vi "Destroy.vi"(8 "error in (no error)":errorcluster, 10 "Wait until done?":bool, 11 "InstrPtr in":refnum<class "InstrPtr.lvclass">) -> (0 "error out":errorcluster, 3 "final Instrument":refnum<class "Instrument.lvclass">)   [LabVIEW 2009, in "InstrPtr.lvclass"]
doc: "Finalizes and destroys this Instrument pointer. You can optionally block if some other process still has a handle."
uses:
  InstrPtr.lvclass
  Instrument/Instrument.lvclass
  InstrPtr.lvclass/InstrPtr.ctl
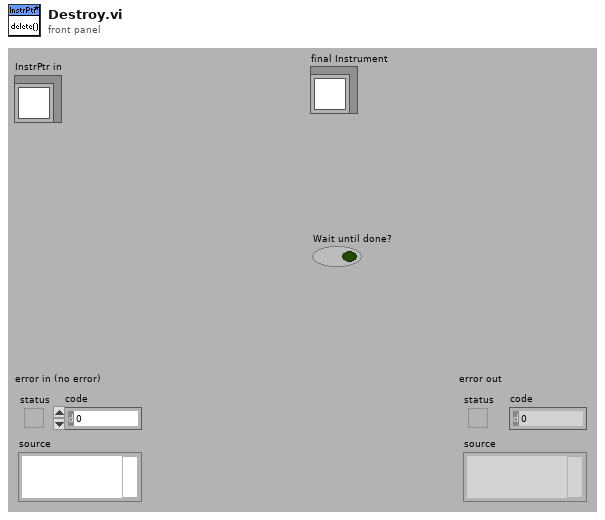
[diagram p1: front panel]
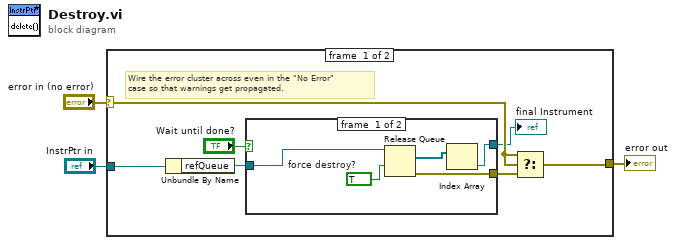
[diagram p0: block diagram]
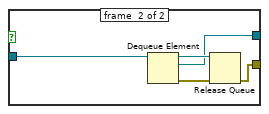
[diagram p2: hidden frame]
diagram:
  n1 = case shown="No Error" "error in (no error)" {
    selector: "error in (no error)" -> [w9 w21]
    tunnel: [w8 w21] -> w2
    tunnel: "InstrPtr in" -> [w10 _]
    frame #0 {
      # "Wire the error cluster across even in the \"No Error\"\ncase so that warnings get propagated."
      n2 = Unbundle By Name(w10) -> ("refQueue"=w6:refnum<queue>)
      n3 = case shown="False" "Wait until done?" {
        tunnel: w6 -> [w13 w20]
        tunnel: [w15 w17] -> w5
        tunnel: [w12 w16] -> w4
        frame #0 {
          w11 = TRUE  # force destroy?
          n4 = Release Queue(queue=w13, force destroy? (F)=w11) -> (remaining elements=w14:refnum<class "Instrument.lvclass">[], error out=w15:errorcluster)  [unwired: 1 in, 1 out]
          n5 = Index Array(array=w14) -> (element=w12:refnum<class "Instrument.lvclass">)  [unwired: 1 in]
        }
        frame #1 {
          n6 = Dequeue Element(queue=w20) -> (queue out=w18:refnum<queue>, element=w16:refnum<class "Instrument.lvclass">, error out=w19:errorcluster)  [unwired: 1 in, 2 out]
          n7 = Release Queue(queue=w18, error in (no error)=w19) -> (error out=w17:errorcluster)  [unwired: 3 out]
        }
      }
      "final Instrument" <- w4
      n8 = Select(t=w9, s=w9, f=w5) -> (s? t:f=w8:errorcluster)
    }
    frame #1 {
    }
  }
  "error out" <- w2
